vi "Cubic Interp.vi"(7 "interp values":dbl[](array[numeric]), 8 "e'":dbl[](array[numeric]), 9 "e":dbl[](array[numeric]), 10 "s'":dbl[](array[numeric]), 11 "s":dbl[](array[numeric])) -> (3 "Array":dbl[][](array[numeric]))   [LabVIEW 2017, in "NI_Robotics_3DKinematics.lvlib"]
uses:
  <vilib>/robotics/Kinematics/Plotting/NI_Robotics_3DKinematics.lvlib
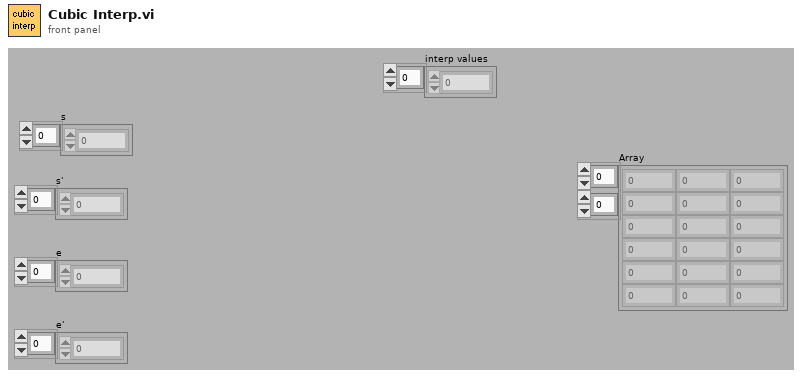
[diagram p1: front panel]
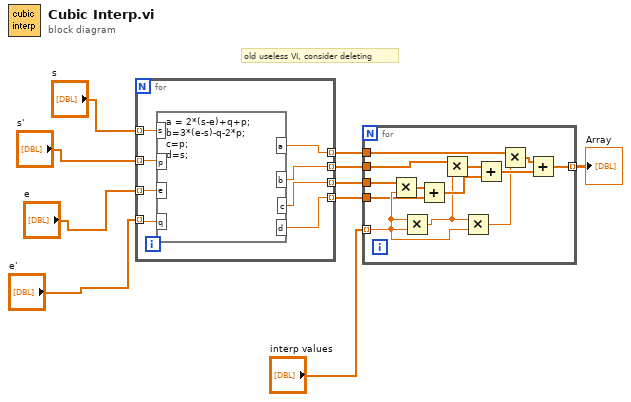
[diagram p0: block diagram]
diagram:
  # "old useless VI, consider deleting"
  n1 = for {
    tunnel: "s" -> [w18] mode=indexing
    tunnel: [w17] -> w9 mode=indexing
    tunnel: [w16] -> w8 mode=indexing
    tunnel: [w15] -> w7 mode=indexing
    tunnel: [w14] -> w6 mode=indexing
    tunnel: "s'" -> [w13] mode=indexing
    tunnel: "e" -> [w12] mode=indexing
    tunnel: "e'" -> [w11] mode=indexing
    n2 = formula code="a = 2*(s-e)+q+p;\nb=3*(e-s)-q-2*p;\nc=p;\nd=s;"("s"=w18, "p"=w13, "e"=w12, "q"=w11) -> ("a"=w17:dbl, "b"=w16:dbl, "c"=w15:dbl, "d"=w14:dbl)
  }
  n3 = for {
    tunnel: "interp values" -> [w30] mode=indexing
    tunnel: w9 -> [w20]
    tunnel: w8 -> [w25]
    tunnel: w7 -> [w31]
    tunnel: w6 -> [w29]
    tunnel: [w19] -> w1 mode=indexing
    n4 = Multiply(x=w31, y=w30) -> (x*y=w28:dbl[])
    n5 = Multiply(x=w30, y=w30) -> (x*y=w24:dbl)
    n6 = Add(x=w28, y=w29) -> (x+y=w27:dbl[])
    n7 = Multiply(x=w25, y=w24) -> (x*y=w22:dbl[])
    n8 = Multiply(x=w24, y=w30) -> (x*y=w23:dbl)
    n9 = Add(x=w22, y=w27) -> (x+y=w26:dbl[])
    n10 = Multiply(x=w20, y=w23) -> (x*y=w21:dbl[])
    n11 = Add(x=w21, y=w26) -> (x+y=w19:dbl[])
  }
  "Array" <- w1
